vi "test_Add Array Comparison .vi"(8 "error in (no error)":errorcluster, 11 "TestCase in":refnum<class "Instrument Addon Scripting API Channels Unit Tests.lvclass">) -> (0 "error out":errorcluster, 3 "TestCase out":refnum<class "Instrument Addon Scripting API Channels Unit Tests.lvclass">)   [LabVIEW 2018, in "Instrument Addon Scripting API Channels Unit Tests.lvclass"]
uses:
  Instrument Addon Scripting API Channels Unit Tests.lvclass
  APIs/Scripting API/TypeDefs/Array Comparison Settings.ctl
  APIs/Scripting API/TypeDefs/Array Element.ctl
  Addon/Addon Shared/Types/Protocol Data Type.ctl
  Addon/Addon Shared/Types/Data Channel Type.ctl
  Instrument Addon Scripting API Channels Unit Tests.lvclass/Instrument Addon Scripting API Channels Unit Tests.ctl
  Addon/Addon Shared/SubVIs/Constants.vi
  <vilib>/NI/NI VeriStand Advanced SysDef API/_SubVIs/SysDef.Search.GUID.vi
  <vilib>/NI/NI VeriStand Advanced SysDef API/_SubVIs/SysDef.Search.GUIDs.vi
  APIs/Scripting API/Channels/Create Data Channel - Array - Comparison.vi
  <vilib>/NI Veristand/Custom Device API/Get Item Property (U16).vi
  <vilib>/NI Veristand/Custom Device API/Get Item Property (String).vi
  <vilib>/addons/_JKI Toolkits/VI Tester/TestCase.llb/TestCase.lvclass
  Instrument Addon Scripting API Test Assets/Instrument Addon Scripting API Test Assets.lvclass
  <vilib>/NI/NI VeriStand Advanced SysDef API/SysDef API/Advanced System Definition.lvlib
  Addon/Addon Shared/Instrument Addon Shared.lvlib
  APIs/Scripting API/Instrument Addon Scripting API.lvlib
  <vilib>/NI Veristand/Custom Device API/Custom Device API.lvlib
  C:/Program Files (x86)/National Instruments/LabVIEW 2018/vi.lib/addons/_JKI Toolkits/VI Tester/TestCase.llb/TestCase.lvclass
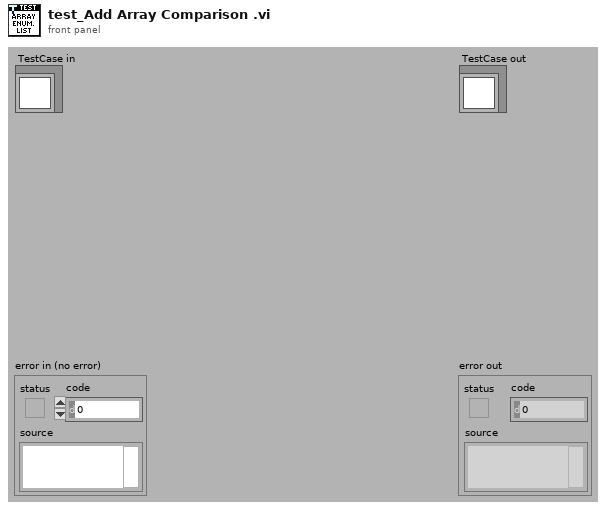
[diagram p1: front panel]
types:
  T1 = typedef "Instrument Addon Scripting API.lvlib/Array Comparison Settings.ctl" = cluster{"Array":T2[], "Expected String(case sensitive)":string, "Delimiter":string}
  T2 = typedef "Instrument Addon Scripting API.lvlib/Array Element.ctl" = cluster{"Name":string, "Default Value":dbl, "Units":string}
  T3 = typedef "Instrument Addon Shared.lvlib/Data Channel Type.ctl" = enum16{"Format", "Comparison", "Type Cast", "Enumerated List"}
  T4 = typedef "Instrument Addon Shared.lvlib/Protocol Data Type.ctl" = enum16{"Single Channel", "Array"}
  T5 = typedef "Custom Device API.lvlib/Custom Device Item Ref.ctl" = u64
  T6 = typedef "Advanced System Definition.lvlib/TreeItem.Info.ctl" = cluster{"Name":string, "Description":string, "GUID":string, "Is Channel":bool, "Channel":T7, "Is Waveform":bool, "Waveform":T9}
  T7 = typedef "Custom Device API.lvlib/Custom Device Channel.ctl" = cluster{"Type":T8, "Units":string, "Default Value":dbl, "Faultable":bool, "Scalable":bool}
  T8 = typedef "Custom Device API.lvlib/Custom Device Channel Type.ctl" = enum16{"Input", "Output"}
  T9 = typedef "Custom Device API.lvlib/Custom Device Waveform.ctl" = cluster{"Data Type":T10, "Units":string}
  T10 = typedef "Custom Device API.lvlib/Custom Device Waveform DataType.ctl" = enum16{"Double", "Complex Double"}
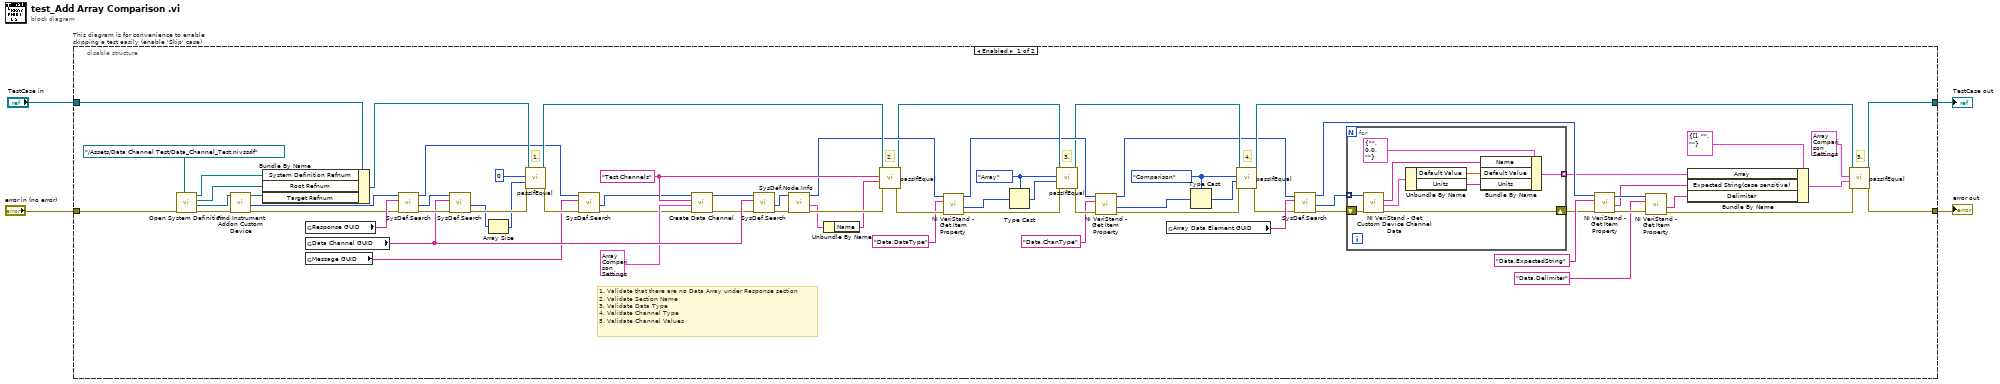
[diagram p0: block diagram]
diagram:
  n1 = disable-structure "This diagram is for convenience to enable skipping a test easily (enable 'Skip' case)" shown="Enabled" {
    disable-tunnel: "TestCase in" -> [w34 w88]
    disable-tunnel: [w50 w86] -> w1
    disable-tunnel: [w51 w87] -> w3
    disable-tunnel: "error in (no error)" -> [w72 w85]
    frame Enabled {
      w11 = Data_Channel_Type."Comparison" ("Channel Type")
      w17 = Protocol_Data_Type."Array" ("Data Type")
      w61 = "Test Channels" ("Name")
      # "4."
      # "3."
      # "5."
      # "2."
      # "1. Validate that there are no Data Array under Response section\n2. Validate Section Name\n3. Validate Data Type\n4. Validate Channel Type\n5. Validate Channel Values"
      # "1."
      n2 = call "Open System Definition.vi"("error in (no error)"=w72, "System Definition File"=path "../Assets/Data Channel Test/Data_Channel_Test.nivssdf") -> ("error out"=w75:errorcluster, "Target Refnum"=w74:refnum<k24>, "Root Refnum"=w36:refnum<k24>, "System Definition Refnum"=w37:refnum<k24>)  [unwired: 6 in]
      n3 = call "Find Instrument Addon Custom Device.vi"("error in"=w75, "target in"=w74) -> ("error out"=w32:errorcluster, "NodeID"=w71:u64, "target out"=w35:refnum<k24>)  [unwired: 7 in]
      n4 = Bundle By Name(cluster=w34, "System Definition Refnum"=w37, "Root Refnum"=w36, "Target Refnum"=w35) -> (w33:refnum<class "Instrument Addon Scripting API Channels Unit Tests.lvclass">)
      n5 = global read "Constants.vi" "Response GUID"() -> (w70:string)
      n6 = global read "Constants.vi" "Data Channel GUID"() -> (w67:string)
      n7 = global read "Constants.vi" "Message GUID"() -> (w29:string)
      n8 = call-poly <vilib>:"SysDef.Search.vi"("error in (no error)"=w32, "GUID"=w70, "nodeID"=w71) -> ("error out"=w68:errorcluster, "Value out"=w69:u64, "nodeID out"=w28:u64)  [unwired: 5 in, 1 out]
      n9 = call-poly <vilib>:"SysDef.Search.vi"("error in (no error)"=w68, "GUID"=w67, "nodeID"=w69) -> ("error out"=w65:errorcluster, "Values Out"=w64:u64[])  [unwired: 5 in, 2 out]
      n10 = Array Size(array=w64) -> (size(s)=w63:i32)
      n11 = call-dynamic "passIfEqual.vi"("error in (no error)"=w65, "y"=w63, "x"=0 ("size(s)"), "TestCase in"=w33) -> ("error out"=w31:errorcluster, "TestCase out"=w66:refnum<class "Instrument Addon Scripting API Channels Unit Tests.lvclass">)  [unwired: 6 in]
      n12 = call-poly <vilib>:"SysDef.Search.vi"("error in (no error)"=w31, "GUID"=w29, "nodeID"=w28) -> ("error out"=w30:errorcluster, "Value out"=w27:u64)  [unwired: 5 in, 2 out]
      n13 = call-poly "Create Data Channel.vi"("Error In"=w30, "Settings"=T1 {"Array"=[{"Name"="Rate", "Default Value"=50.0, "Units"="Hz"}, {"Name"="Wait", "Default Value"=100.0, "Units"="ms"}], "Expected String(case sensitive)"="ExpectedStringExample", "Delimiter"="*"}, "Name"=w61, "Message Refnum In"=w27) -> ("Error Out"=w60:errorcluster, "Message Refnum Out"=w59:T5)  [unwired: 5 in, 1 out]
      n14 = call-poly <vilib>:"SysDef.Search.vi"("error in (no error)"=w60, "GUID"=w67, "nodeID"=w59) -> ("error out"=w58:errorcluster, "Value out"=w24:u64)  [unwired: 5 in, 2 out]
      n15 = call <vilib>:"SysDef.Node.Info.vi"("error in (no error)"=w58, "nodeID"=w24) -> ("error out"=w57:errorcluster, "Item Info"=w56:T6, "nodeID out"=w22:u64)  [unwired: 6 in, 1 out]
      n16 = Unbundle By Name(w56) -> ("Name"=w55:string)
      n17 = call-dynamic "passIfEqual.vi"("error in (no error)"=w57, "y"=w55, "x"=w61, "TestCase in"=w66) -> ("error out"=w23:errorcluster, "TestCase out"=w16:refnum<class "Instrument Addon Scripting API Channels Unit Tests.lvclass">)  [unwired: 6 in]
      n18 = call-poly <vilib>:"NI VeriStand - Get Item Property.vi"("error in (no error)"=w23, "Property Name"="Data.DataType", "Item Ref in"=w22) -> ("error out"=w20:errorcluster, "Value"=w19:u16, "Item Ref out"=w9:T5)  [unwired: 5 in, 1 out]
      n19 = Type Cast(type=w17, x=w19) -> (*(type *) &x=w18:T4)
      n20 = call-dynamic "passIfEqual.vi"("error in (no error)"=w20, "y"=w18, "x"=w17, "TestCase in"=w16) -> ("error out"=w15:errorcluster, "TestCase out"=w8:refnum<class "Instrument Addon Scripting API Channels Unit Tests.lvclass">)  [unwired: 6 in]
      n21 = call-poly <vilib>:"NI VeriStand - Get Item Property.vi"("error in (no error)"=w15, "Property Name"="Data.ChanType", "Item Ref in"=w9) -> ("error out"=w14:errorcluster, "Value"=w13:u16, "Item Ref out"=w6:T5)  [unwired: 5 in, 1 out]
      n22 = global read "Constants.vi" "Array Data Element GUID"() -> (w53:string)
      n23 = Type Cast(type=w11, x=w13) -> (*(type *) &x=w12:T3)
      n24 = call-dynamic "passIfEqual.vi"("error in (no error)"=w14, "y"=w12, "x"=w11, "TestCase in"=w8) -> ("error out"=w10:errorcluster, "TestCase out"=w7:refnum<class "Instrument Addon Scripting API Channels Unit Tests.lvclass">)  [unwired: 6 in]
      n25 = call-poly <vilib>:"SysDef.Search.vi"("error in (no error)"=w10, "GUID"=w53, "nodeID"=w6) -> ("error out"=w54:errorcluster, "Values Out"=w52:u64[], "nodeID out"=w47:u64)  [unwired: 5 in, 1 out]
      n26 = for {
        shift-right: [w76] -> w48
        shift-left: w54 -> [w83]
        tunnel: w52 -> [w84] mode=indexing
        tunnel: [w77] -> w46 mode=indexing
        n27 = call <vilib>:"NI VeriStand - Get Custom Device Channel Data.vi"("error in (no error)"=w83, "Channel Ref in"=w84) -> ("error out"=w76:errorcluster, "Channel"=w80:T7, "Channel Name"=w81:string)  [unwired: 4 in, 3 out]
        n28 = Unbundle By Name(w80) -> ("Default Value"=w78:dbl, "Units"=w79:string)
        n29 = Bundle By Name(cluster=T2 {"Name"="", "Default Value"=0.0, "Units"=""} ("Array Element"), "Name"=w81, "Default Value"=w78, "Units"=w79) -> (w77:T2)
      }
      n30 = call-poly <vilib>:"NI VeriStand - Get Item Property.vi"("error in (no error)"=w48, "Property Name"="Data.ExpectedString", "Item Ref in"=w47) -> ("error out"=w45:errorcluster, "Value"=w38:string, "Item Ref out"=w44:T5)  [unwired: 5 in, 1 out]
      n31 = call-poly <vilib>:"NI VeriStand - Get Item Property.vi"("error in (no error)"=w45, "Property Name"="Data.Delimiter", "Item Ref in"=w44) -> ("error out"=w41:errorcluster, "Value"=w42:string)  [unwired: 5 in, 2 out]
      n32 = Bundle By Name(cluster=T1 {"Array"=[], "Expected String(case sensitive)"="", "Delimiter"=""} ("Settings"), "Array"=w46, "Expected String(case sensitive)"=w38, "Delimiter"=w42) -> (w25:T1)
      n33 = call-dynamic "passIfEqual.vi"("error in (no error)"=w41, "y"=w25, "x"=T1 {"Array"=[{"Name"="Rate", "Default Value"=50.0, "Units"="Hz"}, {"Name"="Wait", "Default Value"=100.0, "Units"="ms"}], "Expected String(case sensitive)"="ExpectedStringExample", "Delimiter"="*"} ("Settings"), "TestCase in"=w7) -> ("error out"=w51:errorcluster, "TestCase out"=w50:refnum<class "Instrument Addon Scripting API Channels Unit Tests.lvclass">)  [unwired: 6 in]
    }
    frame Disabled {
      # "skip test result while test is under development"
      n34 = call <vilib>:"skip.vi"("error in (no error)"=w85, "TestCase in"=w88) -> ("error out"=w87:errorcluster, "TestCase out"=w86:refnum<class "Instrument Addon Scripting API Channels Unit Tests.lvclass">)  [unwired: 8 in]
    }
  }
  "error out" <- w3
  "TestCase out" <- w1
